vi "Teleop.vi"(10 "Match Info":T1={"Autonomous Elapsed Seconds"=0.0, "TeleOp Elapsed Seconds"=0.0, "Disabled Elapsed Seconds"=0.0, "Visited Autonomous"=FALSE, "Visited TeleOp"=FALSE, "Visited Disabled"=FALSE, "Autonomous Settings"={"Autonomous Style"=enum."Independent", "VI Refnum"=refnum}}, 11 "Call Context":T2) -> ()   [LabVIEW 2018]
doc: "This VI is called for each TeleOp packet received from the DS where the robot is not disabled. It is often used to read from the joysticks and update I/O or to update setpoints for timed control loops. It should complete and return within 20 milliseconds or it may miss DS packets."
uses:
  <vilib>/Rock Robotics/WPI/DriverStation/WPI_DriverStationDerivedRobotMode.ctl
  <vilib>/Rock Robotics/WPI/DriverStation/WPI_DriverStationMatch Info.ctl
  <vilib>/Rock Robotics/WPI/Solenoid/WPI_SolenoidValue.ctl
  <vilib>/Rock Robotics/WPI/Utilities/WPI_GetSetVariantRefNum.vi
  Robot Global Data.vi
  <vilib>/Rock Robotics/Network Tables/NT Write Number.vi
  <vilib>/Rock Robotics/Network Tables/NT Write Numeric Array.vi
  <vilib>/Rock Robotics/WPI/Solenoid/WPI_SolenoidSetEnum.vi
  <vilib>/Rock Robotics/Network Tables/NT Write Boolean Array.vi
  <vilib>/Rock Robotics/Network Tables/NT Read Boolean.vi
  <vilib>/Rock Robotics/Network Tables/NT Read Number.vi
panel:
  out "Sample Slider 0":dbl(slide) scale=0.0..5.0
  out "Sample Boolean 1":bool
  out "Sample Boolean 0":bool
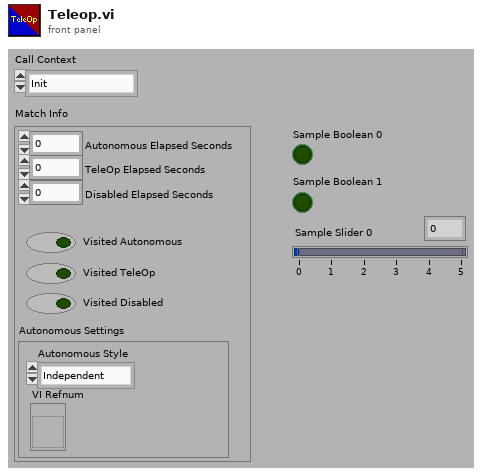
[diagram p1: front panel]
types:
  T1 = typedef "WPI_DriverStationMatch Info.ctl" = cluster{"Autonomous Elapsed Seconds":dbl, "TeleOp Elapsed Seconds":dbl, "Disabled Elapsed Seconds":dbl, "Visited Autonomous":bool, "Visited TeleOp":bool, "Visited Disabled":bool, "Autonomous Settings":cluster{"Autonomous Style":enum16{"Iterative", "Independent"}, "VI Refnum":refnum<vi>}}
  T2 = typedef "WPI_DriverStationDerivedRobotMode.ctl" = enum16{"Init", "Execute", "Stop"}
  T3 = typedef "WPI_SolenoidValue.ctl" = enum16{"Off", "On", "Forward", "Reverse"}
  T4 = typedef "WPI_JoystickDevRef.ctl" = cluster{"Device":T5}
  T5 = typedef "WPI_JoystickDeviceEnum.ctl" = enum16{"USB 0", "USB 1", "USB 2", "USB 3", "USB 4", "USB 5"}
  T6 = typedef "WPI_MotorControlDeviceRef.ctl" = cluster{"DeviceStatus":errorcluster, "Type":T7, "PWM":cluster{"PWM Channel":T8, "DeadBand":T9}, "CAN":cluster{"Device Number":u8, "SetOutput VI Ref":variant, "GetOutput VI Ref":variant, "Enable VI Ref":variant, "Disable VI Ref":variant, "Data":variant}, "Invert":bool, "DIO PWM":cluster{"PWM \"Enable\" Channel":T8, "DIOChannel":T10, "PWM Rate":dbl}}
  T7 = typedef "WPI_MotorControlType.ctl" = enum16{"PWM", "CAN", "DIO PWM"}
  T8 = typedef "FPGA_DIOPWMChannel.ctl" = enum8{"PWM 0", "PWM 1", "PWM 2", "PWM 3", "PWM 4", "PWM 5", "PWM 6", "PWM 7", "PWM 8", "PWM 9", "PWM MXP 0", "PWM MXP 1", "PWM MXP 2", "PWM MXP 3", "PWM MXP 4", "PWM MXP 5", "PWM MXP 6", "PWM MXP 7", "PWM MXP 8", "PWM MXP 9", "Invalid"}
  T9 = typedef "WPI_PWMDeadband.ctl" = cluster{"Name":string, "maxPositivePwm":i32, "minPositivePwm":i32, "centerPwm":i32, "maxNegativePwm":i32, "minNegativePwm":i32, "angularRange":u16}
  T10 = typedef "FPGA_DIOChannel.ctl" = enum8{"DIO 0", "DIO 1", "DIO 2", "DIO 3", "DIO 4", "DIO 5", "DIO 6", "DIO 7", "DIO 8", "DIO 9", "DIO MXP 0", "DIO MXP 1", "DIO MXP 2", "DIO MXP 3", "DIO MXP 4", "DIO MXP 5", "DIO MXP 6", "DIO MXP 7", "DIO MXP 8", "DIO MXP 9", "DIO MXP 10", "DIO MXP 11", "DIO MXP 12", "DIO MXP 13", "DIO MXP 14", "DIO MXP 15", "SPI Port CS1", "SPI Port CS2", "SPI Port CS3", "SPI Port MISO", "SPI Port MOSI", "Invalid"}
  T11 = typedef "WPI_RobotDriveDevRef.ctl" = cluster{"DevStatus":errorcluster, "Motors[]":T6[], "Square Inputs":bool, "Max Output":dbl}
  T12 = typedef "WPI_SolenoidDevRef.ctl" = cluster{"DevStatus":errorcluster, "Pneumatics Control Module":u8, "Forward Solenoid Channel":T13, "Reverse Solenoid Channel":T13}
  T13 = typedef "WPI_SolenoidChannel.ctl" = enum8{"Solenoid 0", "Solenoid 1", "Solenoid 2", "Solenoid 3", "Solenoid 4", "Solenoid 5", "Solenoid 6", "Solenoid 7", "Invalid"}
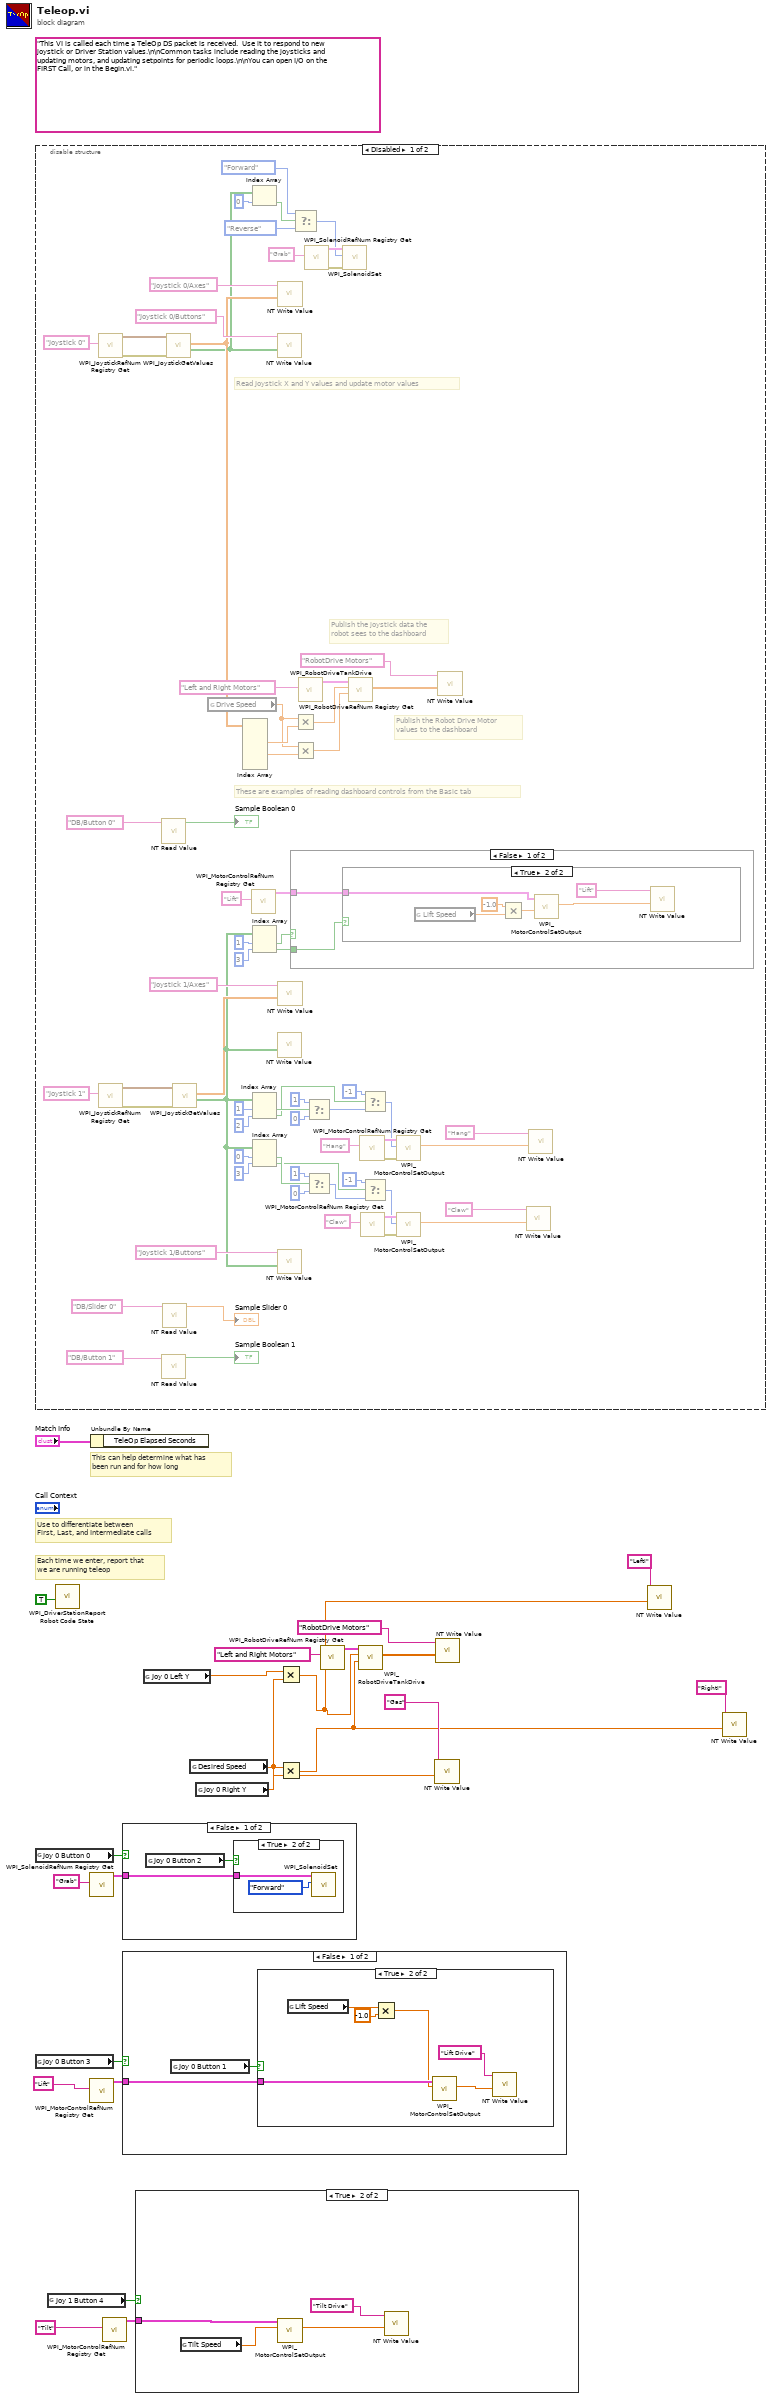
[diagram p0: block diagram]
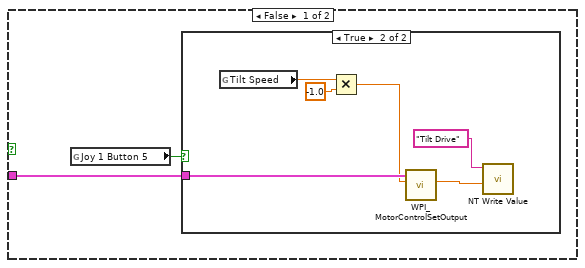
[diagram p2: hidden frame]
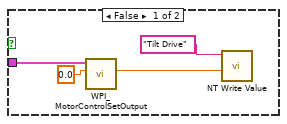
[diagram p3: hidden frame]
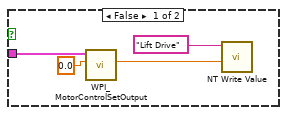
[diagram p4: hidden frame]
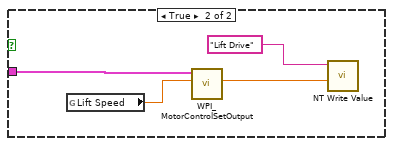
[diagram p5: hidden frame]
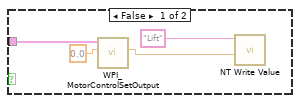
[diagram p6: hidden frame]
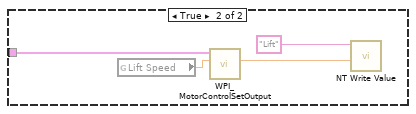
[diagram p7: hidden frame]
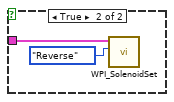
[diagram p10: hidden frame]
diagram:
  (unwired) "This VI is called each time a TeleOp DS packet is received.  Use it to respond to new joystick or Driver Station values.\n\nCommon tasks include reading the joysticks and updating motors, and updating setpoints for periodic loops.\n\nYou can open I/O on the FIRST Call, or in the Begin.vi."
  # "Each time we enter, report that\nwe are running teleop"
  # "Use to differentiate between\nFirst, Last, and Intermediate calls"
  # "This can help determine what has\nbeen run and for how long"
  n1 = disable-structure shown="Disabled" {
    frame Disabled {
      # "These are examples of reading dashboard controls from the Basic tab"
      # "Publish the Robot Drive Motor\nvalues to the dashboard"
      # "Publish the joystick data the\nrobot sees to the dashboard"
      # "Read Joystick X and Y values and update motor values"
      n2 = call <vilib>:"WPI_JoystickRefNum Registry Get.vi"("refnum name"="Joystick 0") -> ("error out"=w38:errorcluster, "JoystickDevRef"=w92:T4)  [unwired: 1 in, 8 out]
      n3 = call <vilib>:"WPI_JoystickRefNum Registry Get.vi"("refnum name"="Joystick 1") -> ("error out"=w75:errorcluster, "JoystickDevRef"=w80:T4)  [unwired: 9 in]
      n4 = call-poly <vilib>:"NT Read Value.vi"("Name"="DB/Button 0" ("refnum name")) -> ("Boolean"=→"Sample Boolean 0":bool)  [unwired: 9 in, 1 out]
      n5 = call-poly <vilib>:"NT Read Value.vi"("Name"="DB/Button 1" ("refnum name")) -> ("Boolean"=→"Sample Boolean 1":bool)  [unwired: 9 in, 1 out]
      n6 = call-poly <vilib>:"NT Read Value.vi"("Name"="DB/Slider 0" ("refnum name")) -> ("Numeric"=→"Sample Slider 0":dbl)  [unwired: 9 in, 1 out]
      n7 = call <vilib>:"WPI_JoystickGetValues.vi"("error in (no error)"=w38, "JoystickDevRef"=w92) -> ("Buttons"=w39:bool[], "Axes"=w89:dbl[])  [unwired: 5 in, 3 out]
      n8 = call <vilib>:"WPI_JoystickGetValues.vi"("error in (no error)"=w75, "JoystickDevRef"=w80) -> ("Buttons"=w29:bool[], "Axes"=w76:dbl[])  [unwired: 5 in, 3 out]
      n9 = global read "Robot Global Data.vi" "Drive Speed"() -> (w31:dbl)
      n10 = Index Array(array=w89) -> (element #2=w45:dbl, element #4=w30:dbl)  [unwired: 6 in, 4 out]
      n11 = call <vilib>:"WPI_MotorControlRefNum Registry Get.vi"("refnum name"="Lift") -> ("MotorControlDevRef"=w25:T6)  [unwired: 9 in, 1 out]
      n12 = Index Array(array=w39, index=0) -> (element=w35:bool)
      n13 = Index Array(array=w29, index #1=1 ("index"), index #2=3 ("index")) -> (element #1=w26:bool, element #2=w24:bool)
      n14 = Index Array(array=w29, index #1=1, index #2=2) -> (element #1=w56:bool, element #2=w48:bool)
      n15 = Index Array(array=w29, index #1=0, index #2=3) -> (element #1=w69:bool, element #2=w62:bool)
      n16 = call-poly <vilib>:"NT Write Value.vi"("Boolean Array"=w39, "Name"="Joystick 0/Buttons") -> ()  [unwired: 9 in, 1 out]
      n17 = call-poly <vilib>:"NT Write Value.vi"("Boolean Array"=w29) -> ()  [unwired: 10 in, 1 out]
      n18 = call-poly <vilib>:"NT Write Value.vi"("Boolean Array"=w29, "Name"="Joystick 1/Buttons") -> ()  [unwired: 9 in, 1 out]
      n19 = call-poly <vilib>:"NT Write Value.vi"("Numeric Array"=w89, "Name"="Joystick 0/Axes") -> ()  [unwired: 9 in, 1 out]
      n20 = call-poly <vilib>:"NT Write Value.vi"("Numeric Array"=w76, "Name"="Joystick 1/Axes") -> ()  [unwired: 9 in, 1 out]
      n21 = case shown="False" w26 {
        tunnel: w25 -> [w95 w110]
        tunnel: w24 -> [w96 _]
        frame False {
          n22 = case shown="True" w96 {
            tunnel: w95 -> [w97 w104]
            frame False {
              n23 = call <vilib>:"WPI_MotorControlSetOutput.vi"("Output"=0.0, "MotorControlDevRef"=w97) -> ("Motor Output"=w99:dbl)  [unwired: 7 in, 2 out]
              n24 = call-poly <vilib>:"NT Write Value.vi"("Numeric"=w99, "Name"="Lift") -> ()  [unwired: 9 in, 1 out]
            }
            frame True {
              n25 = global read "Robot Global Data.vi" "Lift Speed"() -> (w102:dbl)
              n26 = Multiply(x=-1.0, y=w102) -> (x*y=w103:dbl)
              n27 = call <vilib>:"WPI_MotorControlSetOutput.vi"("options"=w103, "MotorControlDevRef"=w104) -> ("Motor Output"=w105:dbl)  [unwired: 7 in, 2 out]
              n28 = call-poly <vilib>:"NT Write Value.vi"("Numeric"=w105, "Name"="Lift") -> ()  [unwired: 9 in, 1 out]
            }
          }
        }
        frame True {
          n29 = global read "Robot Global Data.vi" "Lift Speed"() -> (w109:dbl)
          n30 = call <vilib>:"WPI_MotorControlSetOutput.vi"("Output"=w109, "MotorControlDevRef"=w110) -> ("Motor Output"=w107:dbl)  [unwired: 7 in, 2 out]
          n31 = call-poly <vilib>:"NT Write Value.vi"("Numeric"=w107, "Name"="Lift") -> ()  [unwired: 9 in, 1 out]
        }
      }
      n32 = Select(t=WPI_SolenoidValue."Forward" ("Value"), s=w35, f=WPI_SolenoidValue."Reverse" ("Value")) -> (s? t:f=w33:T3)
      n33 = Multiply(x=w31, y=w45) -> (x*y=w44:dbl)
      n34 = Multiply(x=w31, y=w30) -> (x*y=w32:dbl)
      n35 = call <vilib>:"WPI_RobotDriveRefNum Registry Get.vi"("refnum name"="Left and Right Motors") -> ("RobotDriveDevRef"=w73:T11)  [unwired: 1 in, 9 out]
      n36 = call <vilib>:"WPI_SolenoidRefNum Registry Get.vi"("refnum name"="Grab") -> ("error out"=w40:errorcluster, "SolenoidDevRef"=w41:T12)  [unwired: 9 in]
      n37 = Select(t=1, s=w56, f=0) -> (s? t:f=w50:i32)
      n38 = Select(t=1, s=w69, f=0) -> (s? t:f=w64:i32)
      n39 = call-poly <vilib>:"WPI_SolenoidSet.vi"("error in (no error)"=w40, "Value"=w33, "SolenoidDevRef"=w41) -> ()  [unwired: 7 in, 2 out]
      n40 = call <vilib>:"WPI_RobotDriveTankDrive.vi"("Right axis value"=w32, "Left axis value"=w44, "RobotDriveDevRef"=w73) -> ("Motor Values"=w74:dbl[])  [unwired: 6 in, 2 out]
      n41 = call <vilib>:"WPI_MotorControlRefNum Registry Get.vi"("refnum name"="Hang") -> ("error out"=w58:errorcluster, "MotorControlDevRef"=w59:T6)  [unwired: 9 in]
      n42 = call <vilib>:"WPI_MotorControlRefNum Registry Get.vi"("refnum name"="Claw") -> ("error out"=w71:errorcluster, "MotorControlDevRef"=w72:T6)  [unwired: 9 in]
      n43 = Select(t=-1, s=w48, f=w50) -> (s? t:f=w53:i32)
      n44 = Select(t=-1, s=w62, f=w64) -> (s? t:f=w34:i32)
      n45 = call <vilib>:"WPI_MotorControlSetOutput.vi"("error in (no error)"=w58, "Output"=w53, "MotorControlDevRef"=w59) -> ("Motor Output"=w47:dbl)  [unwired: 6 in, 2 out]
      n46 = call <vilib>:"WPI_MotorControlSetOutput.vi"("error in (no error)"=w71, "Output"=w34, "MotorControlDevRef"=w72) -> ("Motor Output"=w61:dbl)  [unwired: 6 in, 2 out]
      n47 = call-poly <vilib>:"NT Write Value.vi"("Numeric Array"=w74, "Name"="RobotDrive Motors") -> ()  [unwired: 9 in, 1 out]
      n48 = call-poly <vilib>:"NT Write Value.vi"("Numeric"=w61, "Name"="Claw") -> ()  [unwired: 9 in, 1 out]
      n49 = call-poly <vilib>:"NT Write Value.vi"("Numeric"=w47, "Name"="Hang") -> ()  [unwired: 9 in, 1 out]
    }
    frame Enabled {
    }
  }
  n50 = global read "Robot Global Data.vi" "Joy 0 Button 0"() -> (w14:bool)
  n51 = global read "Robot Global Data.vi" "Joy 0 Button 3"() -> (w12:bool)
  n52 = global read "Robot Global Data.vi" "Joy 1 Button 4"() -> (w9:bool)
  n53 = call <vilib>:"WPI_DriverStationReport Robot Code State.vi"("TeleOp"=TRUE ("Autonomous")) -> ()  [unwired: 10 in, 1 out]
  n54 = call <vilib>:"WPI_SolenoidRefNum Registry Get.vi"("refnum name"="Grab") -> ("SolenoidDevRef"=w15:T12)  [unwired: 9 in, 1 out]
  n55 = call <vilib>:"WPI_MotorControlRefNum Registry Get.vi"("refnum name"="Lift") -> ("MotorControlDevRef"=w11:T6)  [unwired: 9 in, 1 out]
  n56 = Unbundle By Name("Match Info") -> ()  [unwired: 1 out]
  n57 = call <vilib>:"WPI_MotorControlRefNum Registry Get.vi"("refnum name"="Tilt") -> ("MotorControlDevRef"=w8:T6)  [unwired: 9 in, 1 out]
  n58 = case shown="False" w14 {
    tunnel: w15 -> [w111 w116]
    frame False {
      n59 = global read "Robot Global Data.vi" "Joy 0 Button 2"() -> (w112:bool)
      n60 = case shown="True" w112 {
        tunnel: w111 -> [_ w113]
        frame False {
        }
        frame True {
          n61 = call-poly <vilib>:"WPI_SolenoidSet.vi"("Value"=WPI_SolenoidValue."Forward", "SolenoidDevRef"=w113) -> ()  [unwired: 8 in, 2 out]
        }
      }
    }
    frame True {
      n62 = call-poly <vilib>:"WPI_SolenoidSet.vi"("Value"=WPI_SolenoidValue."Reverse", "SolenoidDevRef"=w116) -> ()  [unwired: 8 in, 2 out]
    }
  }
  n63 = case shown="False" w12 {
    tunnel: w11 -> [w117 w130]
    frame False {
      n64 = global read "Robot Global Data.vi" "Joy 0 Button 1"() -> (w118:bool)
      n65 = case shown="True" w118 {
        tunnel: w117 -> [w119 w126]
        frame False {
          n66 = call <vilib>:"WPI_MotorControlSetOutput.vi"("Output"=0.0, "MotorControlDevRef"=w119) -> ("Motor Output"=w121:dbl)  [unwired: 7 in, 2 out]
          n67 = call-poly <vilib>:"NT Write Value.vi"("Numeric"=w121, "Name"="Lift Drive") -> ()  [unwired: 9 in, 1 out]
        }
        frame True {
          n68 = global read "Robot Global Data.vi" "Lift Speed"() -> (w125:dbl)
          n69 = Multiply(x=w125, y=-1.0) -> (x*y=w123:dbl)
          n70 = call <vilib>:"WPI_MotorControlSetOutput.vi"("Output"=w123, "MotorControlDevRef"=w126) -> ("Motor Output"=w127:dbl)  [unwired: 7 in, 2 out]
          n71 = call-poly <vilib>:"NT Write Value.vi"("Numeric"=w127, "Name"="Lift Drive") -> ()  [unwired: 9 in, 1 out]
        }
      }
    }
    frame True {
      n72 = global read "Robot Global Data.vi" "Lift Speed"() -> (w129:dbl)
      n73 = call <vilib>:"WPI_MotorControlSetOutput.vi"("Output"=w129, "MotorControlDevRef"=w130) -> ("Motor Output"=w131:dbl)  [unwired: 7 in, 2 out]
      n74 = call-poly <vilib>:"NT Write Value.vi"("Numeric"=w131, "Name"="Lift Drive") -> ()  [unwired: 9 in, 1 out]
    }
  }
  n75 = case shown="True" w9 {
    tunnel: w8 -> [w133 w146]
    frame False {
      n76 = global read "Robot Global Data.vi" "Joy 1 Button 5"() -> (w134:bool)
      n77 = case shown="True" w134 {
        tunnel: w133 -> [w135 w142]
        frame False {
          n78 = call <vilib>:"WPI_MotorControlSetOutput.vi"("Output"=0.0, "MotorControlDevRef"=w135) -> ("Motor Output"=w137:dbl)  [unwired: 7 in, 2 out]
          n79 = call-poly <vilib>:"NT Write Value.vi"("Numeric"=w137, "Name"="Tilt Drive") -> ()  [unwired: 9 in, 1 out]
        }
        frame True {
          n80 = global read "Robot Global Data.vi" "Tilt Speed"() -> (w141:dbl)
          n81 = Multiply(x=w141, y=-1.0) -> (x*y=w139:dbl)
          n82 = call <vilib>:"WPI_MotorControlSetOutput.vi"("Output"=w139, "MotorControlDevRef"=w142) -> ("Motor Output"=w143:dbl)  [unwired: 7 in, 2 out]
          n83 = call-poly <vilib>:"NT Write Value.vi"("Numeric"=w143, "Name"="Tilt Drive") -> ()  [unwired: 9 in, 1 out]
        }
      }
    }
    frame True {
      n84 = global read "Robot Global Data.vi" "Tilt Speed"() -> (w145:dbl)
      n85 = call <vilib>:"WPI_MotorControlSetOutput.vi"("Output"=w145, "MotorControlDevRef"=w146) -> ("Motor Output"=w147:dbl)  [unwired: 7 in, 2 out]
      n86 = call-poly <vilib>:"NT Write Value.vi"("Numeric"=w147, "Name"="Tilt Drive") -> ()  [unwired: 9 in, 1 out]
    }
  }
  n87 = global read "Robot Global Data.vi" "Joy 0 Left Y"() -> (w7:dbl)
  n88 = global read "Robot Global Data.vi" "Desired Speed"() -> (w6:dbl)
  n89 = global read "Robot Global Data.vi" "Joy 0 Right Y"() -> (w21:dbl)
  n90 = Multiply(x=w7, y=w6) -> (x*y=w1:dbl)
  n91 = Multiply(x=w6, y=w21) -> (x*y=w2:dbl)
  n92 = call <vilib>:"WPI_RobotDriveRefNum Registry Get.vi"("refnum name"="Left and Right Motors") -> ("RobotDriveDevRef"=w17:T11)  [unwired: 1 in, 9 out]
  n93 = call <vilib>:"WPI_RobotDriveTankDrive.vi"("Right axis value"=w2, "Left axis value"=w1, "RobotDriveDevRef"=w17) -> ("Motor Values"=w18:dbl[])  [unwired: 6 in, 2 out]
  n94 = call-poly <vilib>:"NT Write Value.vi"("Numeric"=w6, "Name"="Gas") -> ()  [unwired: 9 in, 1 out]
  n95 = call-poly <vilib>:"NT Write Value.vi"("Numeric Array"=w18, "Name"="RobotDrive Motors") -> ()  [unwired: 9 in, 1 out]
  n96 = call-poly <vilib>:"NT Write Value.vi"("Numeric"=w1, "Name"="LeftI") -> ()  [unwired: 9 in, 1 out]
  n97 = call-poly <vilib>:"NT Write Value.vi"("Numeric"=w2, "Name"="RightI") -> ()  [unwired: 9 in, 1 out]
